vi "Read INodeFactory.vi"(11 "Search in":refnum<class "Search.lvclass">) -> (2 "INodeFactory.lvclass":refnum<class "INodeFactory.lvclass">, 3 "Search out":refnum<class "Search.lvclass">)   [LabVIEW 2016, in "Search.lvclass"]
uses:
  Search.lvclass
  INodeFactory/INodeFactory.lvclass
  Search.lvclass/Search.ctl
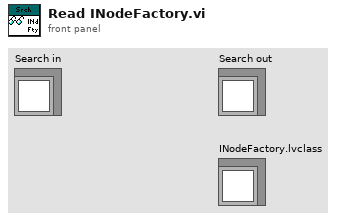
[diagram p1: front panel]
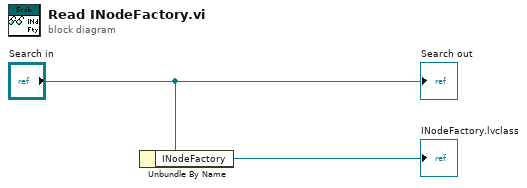
[diagram p0: block diagram]
diagram:
  n1 = Unbundle By Name("Search in") -> ("INodeFactory"=→"INodeFactory.lvclass":refnum<class "INodeFactory.lvclass">)
  "Search out" <- "Search in"
